vi "质控报警信息存储 (子VI).vi"   [LabVIEW 2016, in "质控单元.lvlib"]
uses:
  <vilib>/ptbypt/NI_PtbyPt.lvlib
types:
  T1 = cluster{"时间标识":timestamp, "设备":string, "日志信息":string}
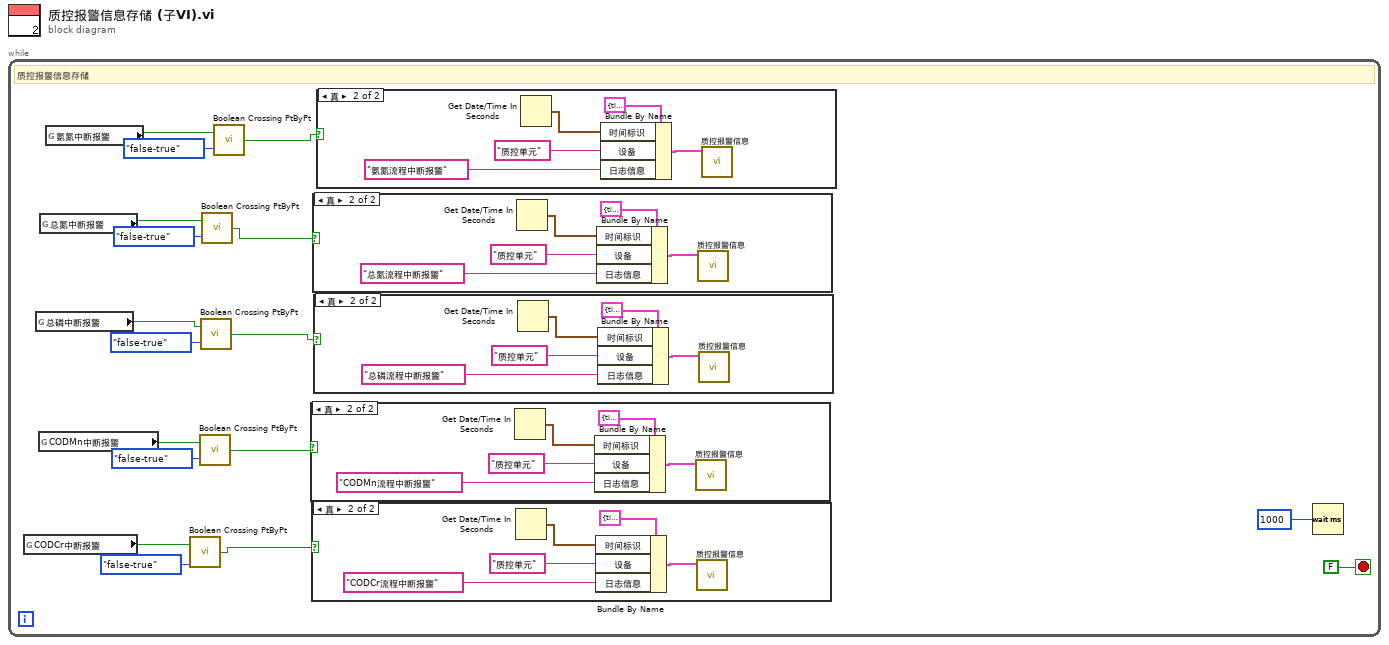
[diagram p0: block diagram]
diagram:
  n1 = while {
    stop <- FALSE stop-if-true
    # "质控报警信息存储"
    n2 = global read "质控中断报警全局.vi" "CODCr中断报警"() -> (w7:bool)
    n3 = global read "质控中断报警全局.vi" "总磷中断报警"() -> (w11:bool)
    n4 = global read "质控中断报警全局.vi" "CODMn中断报警"() -> (w9:bool)
    n5 = global read "质控中断报警全局.vi" "总氮中断报警"() -> (w13:bool)
    n6 = global read "质控中断报警全局.vi" "氨氮中断报警"() -> (w15:bool)
    n7 = call <vilib>:"Boolean Crossing PtByPt.vi"("direction"=enum16{"either", "false-true", "true-false"}."false-true", "input"=w7) -> ("crossing"=w1:bool)  [unwired: 1 in]
    n8 = call <vilib>:"Boolean Crossing PtByPt.vi"("direction"=enum16{"either", "false-true", "true-false"}."false-true", "input"=w9) -> ("crossing"=w2:bool)  [unwired: 1 in]
    n9 = call <vilib>:"Boolean Crossing PtByPt.vi"("direction"=enum16{"either", "false-true", "true-false"}."false-true", "input"=w11) -> ("crossing"=w3:bool)  [unwired: 1 in]
    n10 = call <vilib>:"Boolean Crossing PtByPt.vi"("direction"=enum16{"either", "false-true", "true-false"}."false-true", "input"=w13) -> ("crossing"=w4:bool)  [unwired: 1 in]
    n11 = call <vilib>:"Boolean Crossing PtByPt.vi"("direction"=enum16{"either", "false-true", "true-false"}."false-true", "input"=w15) -> ("crossing"=w5:bool)  [unwired: 1 in]
    n12 = case shown="真" w2 {
      frame False {
      }
      frame True {
        n13 = Get Date/Time In Seconds() -> (seconds since 1Jan1904=w27:timestamp)
        n14 = Bundle By Name(cluster=T1 {"时间标识"=timestamp(0 s since 1904-01-01), "设备"="", "日志信息"=""} ("data in"), "时间标识"=w27, "设备"="质控单元", "日志信息"="CODMn流程中断报警") -> (w23:T1)
        n15 = call "质控报警信息.vi"("data in"=w23) -> ()  [unwired: 10 in, 1 out]
      }
    }
    n16 = case shown="真" w1 {
      frame False {
      }
      frame True {
        n17 = Get Date/Time In Seconds() -> (seconds since 1Jan1904=w22:timestamp)
        n18 = Bundle By Name(cluster=T1 {"时间标识"=timestamp(0 s since 1904-01-01), "设备"="", "日志信息"=""} ("data in"), "时间标识"=w22, "设备"="质控单元", "日志信息"="CODCr流程中断报警") -> (w18:T1)
        n19 = call "质控报警信息.vi"("data in"=w18) -> ()  [unwired: 10 in, 1 out]
      }
    }
    n20 = case shown="真" w4 {
      frame False {
      }
      frame True {
        n21 = Get Date/Time In Seconds() -> (seconds since 1Jan1904=w37:timestamp)
        n22 = Bundle By Name(cluster=T1 {"时间标识"=timestamp(0 s since 1904-01-01), "设备"="", "日志信息"=""} ("data in"), "时间标识"=w37, "设备"="质控单元", "日志信息"="总氮流程中断报警") -> (w33:T1)
        n23 = call "质控报警信息.vi"("data in"=w33) -> ()  [unwired: 10 in, 1 out]
      }
    }
    n24 = case shown="真" w3 {
      frame False {
      }
      frame True {
        n25 = Get Date/Time In Seconds() -> (seconds since 1Jan1904=w32:timestamp)
        n26 = Bundle By Name(cluster=T1 {"时间标识"=timestamp(0 s since 1904-01-01), "设备"="", "日志信息"=""} ("data in"), "时间标识"=w32, "设备"="质控单元", "日志信息"="总磷流程中断报警") -> (w28:T1)
        n27 = call "质控报警信息.vi"("data in"=w28) -> ()  [unwired: 10 in, 1 out]
      }
    }
    n28 = case shown="真" w5 {
      frame False {
      }
      frame True {
        n29 = Get Date/Time In Seconds() -> (seconds since 1Jan1904=w42:timestamp)
        n30 = Bundle By Name(cluster=T1 {"时间标识"=timestamp(0 s since 1904-01-01), "设备"="", "日志信息"=""} ("data in"), "时间标识"=w42, "设备"="质控单元", "日志信息"="氨氮流程中断报警") -> (w38:T1)
        n31 = call "质控报警信息.vi"("data in"=w38) -> ()  [unwired: 10 in, 1 out]
      }
    }
    n32 = Wait (ms)(milliseconds to wait=u32 1000 ("等待时间（毫秒）")) -> ()  [unwired: 1 out]
  }
